vi "X_Write to XML File(string).vi"(4 "File Extension (xml)":string="xml", 5 "Pattern (*.xml;*.XML)":string="*.xml;*.XML", 6 "default name":string, 7 "Prompt":string="Select Path to XML File", 8 "error in (no error)":errorcluster, 10 "XML Input":string, 11 "XML File Start Path":path) -> (0 "error out":errorcluster, 1 "cancelled":bool, 2 "XML String":string, 3 "XML File Path":path)   [LabVIEW 2021, in "Files.lvlib"]
doc: "Writes a text string of XML data with accompanying header tags to a text file. Wire data to the <B>XML Input</B> input to determine the polymorphic instance to use or manually select the instance. All XML data must follow the standard LabVIEW XML schema."
uses:
  Files.lvlib
panel:
  in  "Standalone? (T)":bool=TRUE
  in  "XML Encoding":string
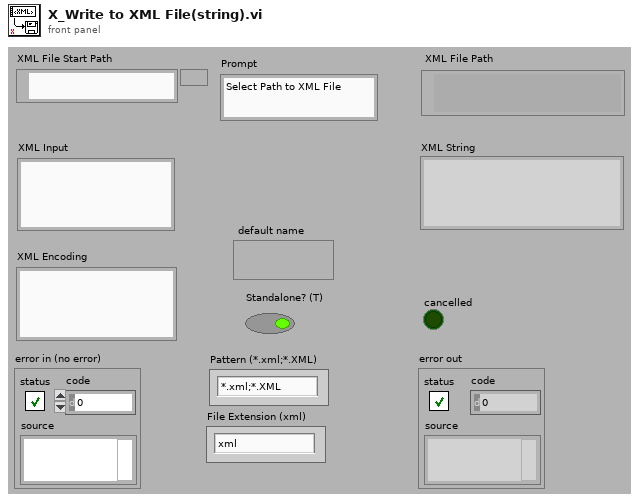
[diagram p1: front panel]
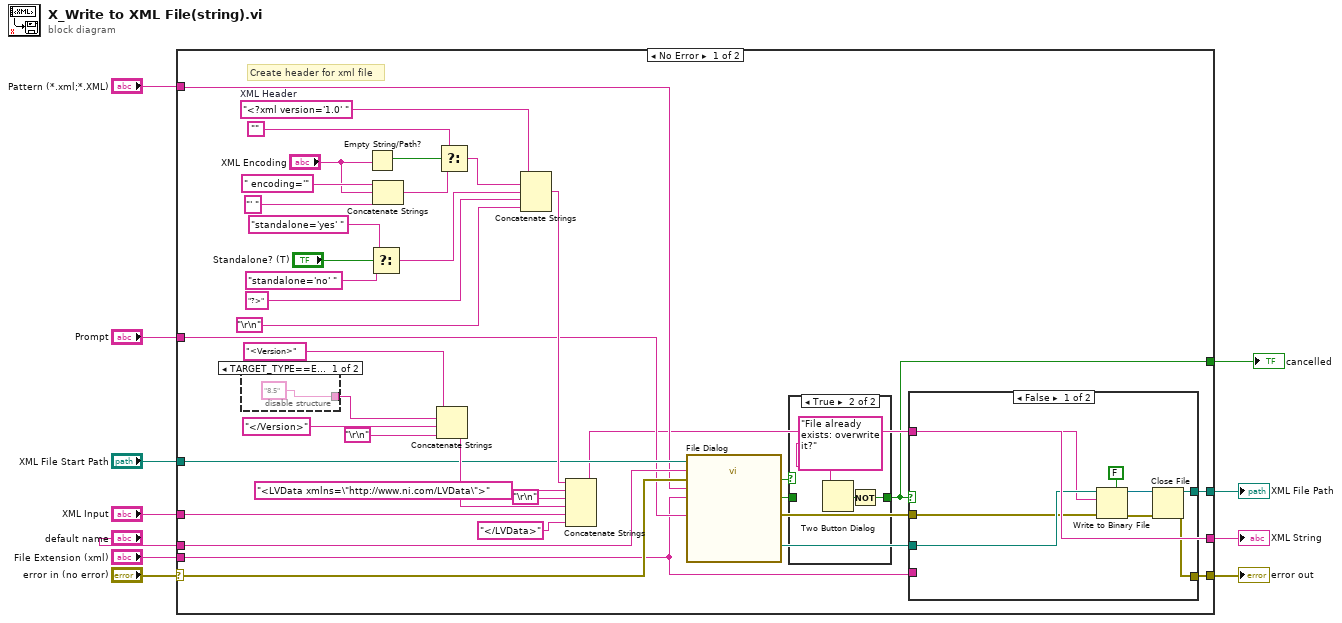
[diagram p0: block diagram]
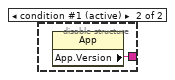
[diagram p4: hidden frame]
diagram:
  n1 = case shown="No Error" "error in (no error)" {
    selector: "error in (no error)" -> [w21 w66]
    tunnel: [w27 w66] -> w10
    tunnel: "XML Input" -> [w34 w65]
    tunnel: [w16 w65] -> w8
    tunnel: [w26 w64] -> w7
    tunnel: "XML File Start Path" -> [w23 w64]
    tunnel: "default name" -> [w22 _]
    tunnel: "Prompt" -> [w19 _]
    tunnel: "Pattern (*.xml;*.XML)" -> [w20 _]
    tunnel: "File Extension (xml)" -> [w15 _]
    tunnel: [w12 _] -> w1
    frame No Error {
      w49 = "<?xml version='1.0' "  # XML Header
      # "Create header for xml file"
      n2 = disable-structure shown="TARGET_TYPE==Embedded||TARGET_TYPE==PocketPC" {
        disable-tunnel: ["8.5" ("App.Version") w63] -> w32
        frame condition #0 {
        }
        frame condition #1 (active) {
          n3 = property class="App"() -> ("App.Version"=w63:string)  [unwired: 2 in, 2 out]
        }
      }
      n4 = Empty String/Path?(string/path="XML Encoding") -> (empty?=w41:bool)
      n5 = Select(t="standalone='yes' " ("Substring"), s="Standalone? (T)", f="standalone='no' " ("Substring")) -> (s? t:f=w35:string)
      n6 = Concatenate Strings(" encoding='", "XML Encoding", "' " ("Substring")) -> (w40:string)
      n7 = Concatenate Strings("<Version>", w32, "</Version>", "\r\n") -> (w29:string)
      n8 = Select(t="", s=w41, f=w40) -> (s? t:f=w38:string)
      n9 = Concatenate Strings(w49, w38, w35, "?>" ("Substring"), "\r\n") -> (w46:string)
      n10 = Concatenate Strings(w46, "<LVData xmlns=\"http://www.ni.com/LVData\">" ("Substring"), "\r\n", w29, w34, "</LVData>" ("Substring")) -> (w16:string)
      n11 = call "File Dialog"("start path"=w23, "prompt"=w19, "default name"=w22, "error in"=w21, "pattern (all files)"=w20, "pattern label"=w15) -> ("selected path"=w18:path, "exists"=w14:bool, "cancelled"=w13:bool, "error out"=w17:errorcluster)  [unwired: 6 in]
      n12 = case shown="True" w14 {
        tunnel: w13 -> [w50 _]
        tunnel: [w50 w51] -> w12
        frame False {
        }
        frame True {
          n13 = Two Button Dialog(message="File already exists: overwrite it?") -> (T button?=w52:bool)  [unwired: 2 in]
          n14 = Not(x=w52) -> (.not. x?=w51:bool)
        }
      }
      n15 = case shown="False" w12 {
        tunnel: [w60 _] -> w27
        tunnel: [w58 _] -> w26
        tunnel: w18 -> [w56 _]
        tunnel: w17 -> [w55 _]
        tunnel: w16 -> [w54 _]
        tunnel: w15 -> [_ _]
        frame False {
          n16 = Write to Binary File(file (use dialog)=w56, data=w54, error in=w55, 5:FALSE ("prepend array or string size? (T)")) -> (refnum out=w59:refnum<file>, error out=w61:errorcluster)  [unwired: 3 out]
          n17 = Close File(refnum=w59, error in=w61) -> (path=w58:path, error out=w60:errorcluster)
        }
        frame True {
        }
      }
    }
    frame Error {
    }
  }
  "error out" <- w10
  "XML String" <- w8
  "XML File Path" <- w7
  "cancelled" <- w1
